vi "Save File Configuration for Order Waveform.vi"() -> (0 "Cancel 2":bool, 2 "Path":path, 3 "binary?":bool)   [LabVIEW 2017]
panel:
  in  "Cancel":bool
  in  "OK":bool
  in  "spreadsheet file":bool
  in  "Save File Path":path
  in  "binary file":bool
  # "Select File Format"
  # "NOTE: The saved binary file can be opened with Read Waveform From File.vi at Waveform File I/O palette"
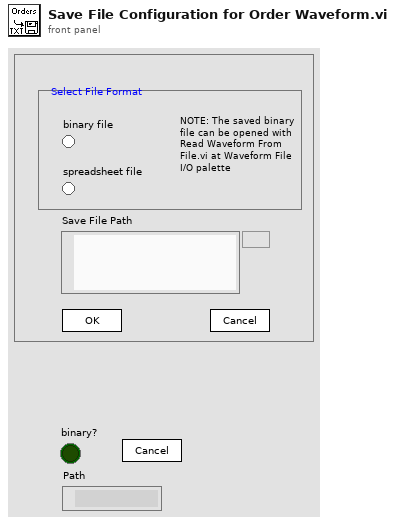
[diagram p1: front panel]
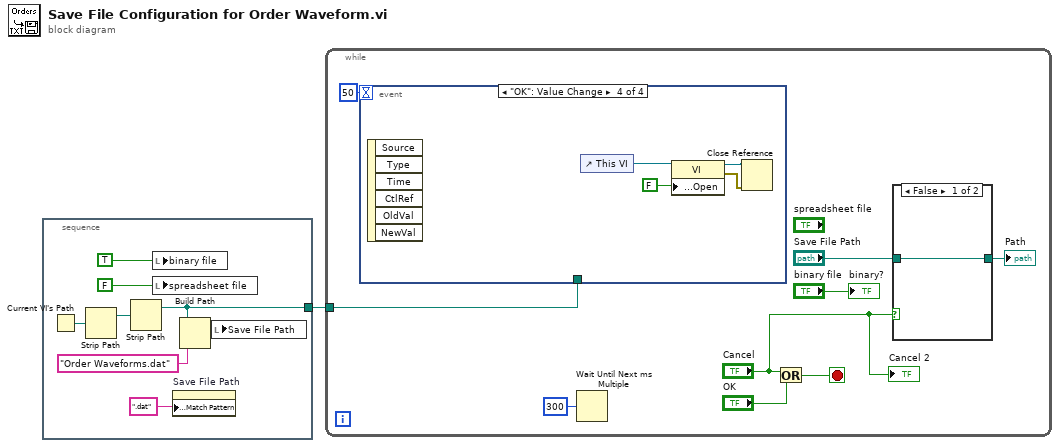
[diagram p0: block diagram]
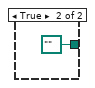
[diagram p2: hidden frame]
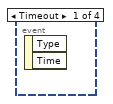
[diagram p3: hidden frame]
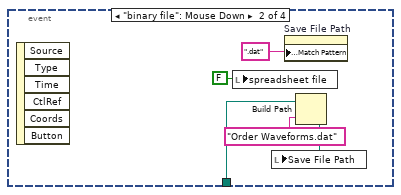
[diagram p4: hidden frame]
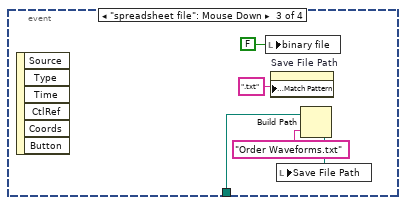
[diagram p5: hidden frame]
diagram:
  n1 = stacked-sequence {
    tunnel: [w3] -> w1
    frame #0 {
      n2 = Current VI's Path() -> (path=w7:path)
      n3 = Strip Path(path=w7) -> (stripped path=w8:path)  [unwired: 1 out]
      n4 = Strip Path(path=w8) -> (stripped path=w3:path)  [unwired: 1 out]
      n5 = local write "binary file"(TRUE ("binary file")) -> ()
      n6 = local write "spreadsheet file"(FALSE ("binary file")) -> ()
      n7 = property on="Save File Path" class="Path"("Browse Options:Match Pattern"=".dat") -> ()  [unwired: 2 in, 2 out]
      n8 = Build Path(base path=w3, name or relative path="Order Waveforms.dat") -> (appended path=w9:path)
      n9 = local write "Save File Path"(w9) -> ()
    }
  }
  n10 = while {
    tunnel: w1 -> [w14]
    stop <- w16 stop-if-true
    n11 = event shown="[3] \"OK\": Value Change" {
      selector: _ -> [_ _ _ _]
      dyn-events: _ -> [_ _ _ _]
      timeout: 50 -> [_ _ _ _]
      tunnel: w14 -> [_ w24 w26 _]
      event Timeout {
        n12 = event-data() -> ()  [unwired: 1 in, 2 out]
      }
      event "binary file": Mouse Down {
        n13 = event-data() -> ()  [unwired: 1 in, 6 out]
        n14 = local write "spreadsheet file"(FALSE ("spreadsheet file")) -> ()
        n15 = property on="Save File Path" class="Path"("Browse Options:Match Pattern"=".dat") -> ()  [unwired: 2 in, 2 out]
        n16 = Build Path(base path=w24, name or relative path="Order Waveforms.dat") -> (appended path=w23:path)
        n17 = local write "Save File Path"(w23) -> ()
      }
      event "spreadsheet file": Mouse Down {
        n18 = event-data() -> ()  [unwired: 1 in, 6 out]
        n19 = local write "binary file"(FALSE ("binary file")) -> ()
        n20 = property on="Save File Path" class="Path"("Browse Options:Match Pattern"=".txt") -> ()  [unwired: 2 in, 2 out]
        n21 = Build Path(base path=w26, name or relative path="Order Waveforms.txt") -> (appended path=w28:path)
        n22 = local write "Save File Path"(w28) -> ()
      }
      event "OK": Value Change {
        n23 = event-data() -> ()  [unwired: 1 in, 6 out]
        n24 = control-ref of="This VI"() -> (w31:refnum<vi>)
        n25 = property class="VI"(reference=w31, "Front Panel Window:Open"=FALSE) -> (reference out=w33:refnum<vi>, error out=w32:errorcluster)  [unwired: 1 in]
        n26 = Close Reference(reference=w33, error in (no error)=w32) -> ()  [unwired: 1 out]
      }
    }
    n27 = Wait Until Next ms Multiple(millisecond multiple=u32 300) -> ()  [unwired: 1 out]
    n28 = Or(x="Cancel", y="OK") -> (x .or. y?=w16:bool)
    n29 = case shown="False" "Cancel" {
      tunnel: "Save File Path" -> [w19 _]
      tunnel: [w19 path "" ("Save File Path")] -> w12
      frame False {
      }
      frame True {
      }
    }
    "Path" <- w12
    "binary?" <- "binary file"
    "Cancel 2" <- "Cancel"
  }
